vi "tinhhuongdichuyen.vi"(8 "dy":dbl, 11 "dx":dbl) -> (3 "phi":dbl)   [LabVIEW 2019]
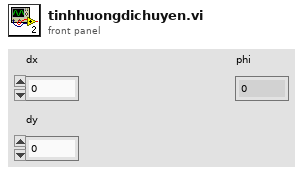
[diagram p1: front panel]
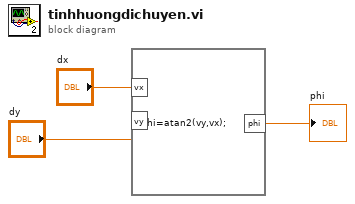
[diagram p0: block diagram]
diagram:
  n1 = formula code="phi=atan2(vy,vx);"("vx"="dx", "vy"="dy") -> ("phi"=→"phi":dbl)
